vi "PCO_DescriptionEx.vi"() -> (0 "PCO_DescriptionEx":cluster{"wSize":u16}, 1 "PCO_DescriptionEx_Raw":cluster{"wSize":u16}, 2 "Length":u16, 3 "Raw_Length":u16)   [LabVIEW 2020, in "SDK.lvlib" / "Structures.lvlib"]
doc: "Use this template to build a VI to use as a subVI."
uses:
  Structures.lvlib
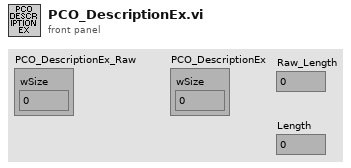
[diagram p1: front panel]
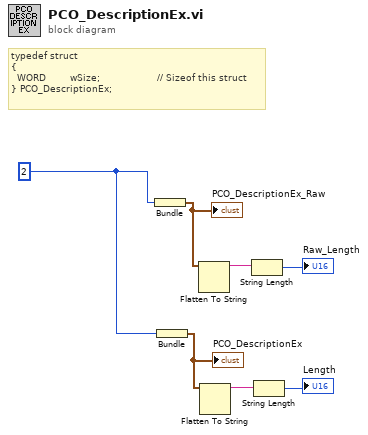
[diagram p0: block diagram]
diagram:
  w1 = u16 2 ("wSize")
  # "typedef struct\n{\n  WORD        wSize;                   // Sizeof this struct\n} PCO_DescriptionEx;"
  n1 = Bundle("wSize"=w1) -> (w7:cluster{"wSize":u16})  [unwired: 1 in]
  "PCO_DescriptionEx_Raw" <- w7
  n2 = Bundle("wSize"=w1) -> (w2:cluster{"wSize":u16})  [unwired: 1 in]
  "PCO_DescriptionEx" <- w2
  n3 = Flatten To String(anything=w7) -> (data string=w5:string)  [unwired: 3 in, 2 out]
  n4 = Flatten To String(anything=w2) -> (data string=w6:string)  [unwired: 3 in, 2 out]
  n5 = String Length(string=w5) -> (length=→"Raw_Length":i32)
  n6 = String Length(string=w6) -> (length=→"Length":i32)
